vi "Module Stopped.vi"(8 "error in":errorcluster) -> (0 "error out":errorcluster)   [LabVIEW 2015, in "Generic Module Library.lvlib" / "Template G_Module.lvlib"]
uses:
  Template G_Module.lvlib
  Private Controls/Event Item.ctl
  Broadcast Support/Broadcast Actions.ctl
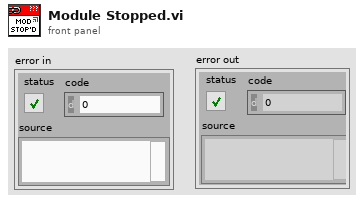
[diagram p1: front panel]
types:
  T1 = typedef "Generic Module Library.lvlib/Template G_Module.lvlib/Broadcast Actions.ctl" = enum16{"Create", "Get", "Destroy"}
  T2 = typedef "Generic Module Library.lvlib/Template G_Module.lvlib/Event Item.ctl" = cluster{"Event Data":variant}
  T3 = typedef "Generic Module Library.lvlib/Template G_Module.lvlib/Broadcast List.ctl" = cluster{"Module Started":refnum<user-event>, "Module Error":refnum<user-event>, "Module Pong":refnum<user-event>, "Module Status":refnum<user-event>, "Module Stopping":refnum<user-event>, "Module Stopped":refnum<user-event>, "Module Reinitialized":refnum<user-event>}
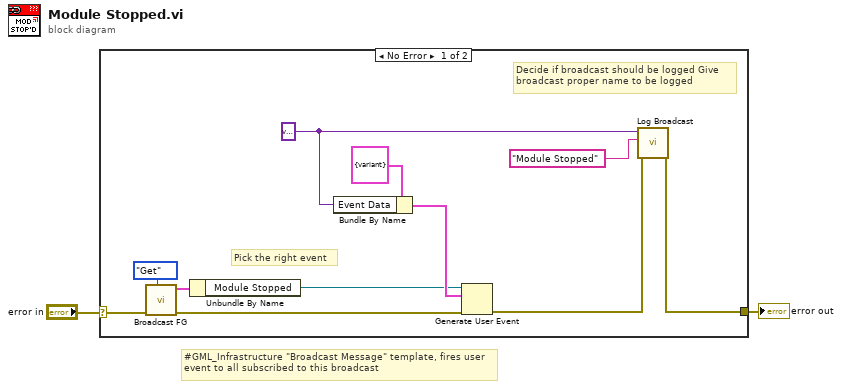
[diagram p0: block diagram]
diagram:
  # "#GML_Infrastructure \"Broadcast Message\" template, fires user event to all subscribed to this broadcast"
  n1 = case shown="No Error" "error in" {
    selector: "error in" -> [w8 w14]
    tunnel: [w6 w14] -> w2
    frame No Error {
      w5 = variant ("Event Data")
      # "Decide if broadcast should be logged Give broadcast proper name to be logged"
      # "Pick the right event"
      n2 = call "Broadcast FG.vi"("Broadcast Actions"=Broadcast_Actions."Get", "error in"=w8) -> ("error out"=w13:errorcluster, "Broadcast List"=w9:T3)  [unwired: 8 in]
      n3 = Unbundle By Name(w9) -> ("Module Stopped"=w4:refnum<user-event>)
      n4 = Bundle By Name(cluster=T2 {"Event Data"=variant} ("Broadcast Item"), "Event Data"=w5) -> (w11:T2)
      n5 = Generate User Event(user event=w4, event data cluster=w11, error in=w13) -> (error out=w7:errorcluster)  [unwired: 1 in, 1 out]
      n6 = call "Log Broadcast.vi"("error in"=w7, "Broadcast Name"="Module Stopped", "Message Data In"=w5) -> ("error out"=w6:errorcluster)  [unwired: 8 in]
    }
    frame Error {
    }
  }
  "error out" <- w2
